vi "Inspect omv.vi"() -> ()   [LabVIEW 2013]
uses:
  <vilib>/Analysis/polynomials.llb/Unique Numbers and Multiplicity (DBL).vi
  <vilib>/Utility/file.llb/Read From Spreadsheet File (string).vi
  <vilib>/Analysis/NI_AALPro.lvlib
panel:
  in  "Open (*.omv)":path
  in  "Tab Control":enum32{"Plot", "VARS"}(tab)
  out "Waveform Graph":dbl[][](graph)
  in  "VAR":u16(ring) items=["XHV"]
  out "min":dbl
  out "max":dbl
  out "Number":i32
  out "Unique":i32
  out "Step size (average)":dbl
  out "VARS":string[](array[string])
  out "Values":string[][](array[string])
  in  "stop":bool
  # "Inspect"
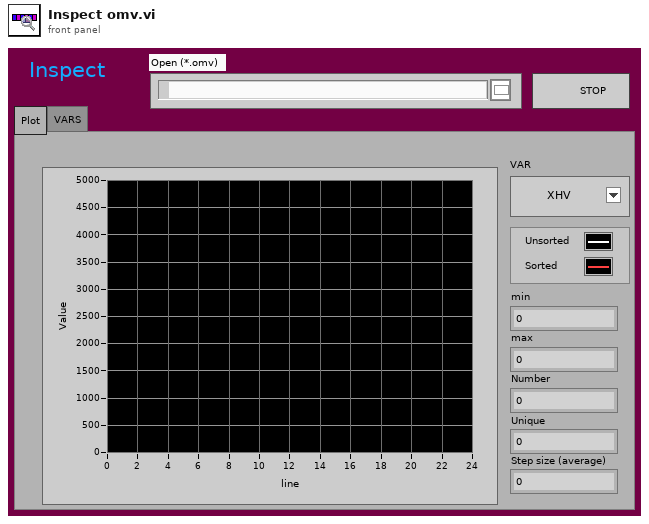
[diagram p1: front panel]
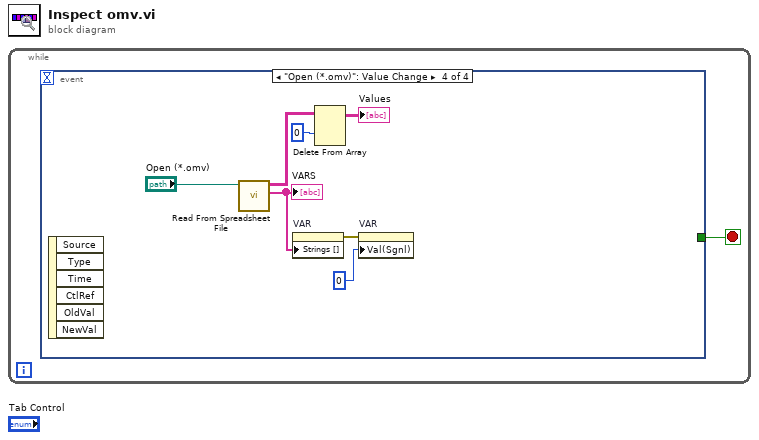
[diagram p0: block diagram]
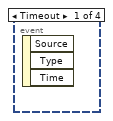
[diagram p2: hidden frame]
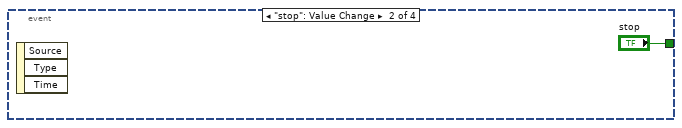
[diagram p3: hidden frame]
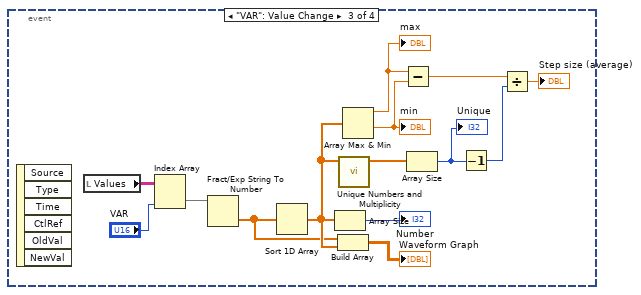
[diagram p4: hidden frame]
diagram:
  n1 = while {
    stop <- w1 stop-if-true
    n2 = event shown="[3] \"Open (*.omv)\": Value Change" {
      selector: _ -> [_ _ _ _]
      dyn-events: _ -> [_ _ _ _]
      timeout: _ -> [_ _ _ _]
      tunnel: [_ "stop" _ _] -> w1
      event Timeout {
        n3 = event-data() -> ()  [unwired: 1 in, 3 out]
      }
      event "stop": Value Change {
        n4 = event-data() -> ()  [unwired: 1 in, 3 out]
      }
      event "VAR": Value Change {
        n5 = event-data() -> ()  [unwired: 1 in, 6 out]
        n6 = local read "Values"() -> (w16:string[][])
        n7 = Index Array(array=w16, index (col)="VAR") -> (element=w3:string[])  [unwired: 1 in]
        n8 = Fract/Exp String To Number(string=w3) -> (number=w4:dbl[])  [unwired: 3 in, 1 out]
        n9 = Sort 1D Array(array=w4) -> (sorted array=w9:dbl[])
        n10 = Array Size(array=w9) -> (size(s)=→"Number":i32)
        n11 = Build Array(w4, w9) -> (→"Waveform Graph":dbl[][])
        n12 = call-poly <vilib>:"Unique Numbers and Multiplicity.vi"("Numbers"=w9) -> ("Unique Numbers"=w8:dbl[])  [unwired: 8 in, 2 out]
        n13 = Array Max & Min(array=w9) -> (max value=w13:dbl, min value=w7:dbl)  [unwired: 2 out]
        "max" <- w13
        "min" <- w7
        n14 = Subtract(x=w13, y=w7) -> (x-y=w12:dbl)
        n15 = Array Size(array=w8) -> (size(s)=w6:i32)
        "Unique" <- w6
        n16 = Decrement(x=w6) -> (x-1=w5:i32)
        n17 = Divide(x=w12, y=w5) -> (x/y=→"Step size (average)":dbl)
      }
      event "Open (*.omv)": Value Change {
        n18 = event-data() -> ()  [unwired: 1 in, 6 out]
        n19 = call-poly <vilib>:"Read From Spreadsheet File.vi"("file path (dialog if empty)"="Open (*.omv)") -> ("first row"=w20:string[], "all rows"=w22:string[][])  [unwired: 6 in, 3 out]
        "VARS" <- w20
        n20 = property on="VAR" class="Ring (strict)"("Strings []"=w20) -> (error out=w18:errorcluster)  [unwired: 2 in, 1 out]
        n21 = Delete From Array(array=w22, index (row)=0) -> (array with subset deleted=→"Values":string[][])  [unwired: 2 in, 1 out]
        n22 = property on="VAR" class="Ring (strict)"(error in=w18, "Val(Sgnl)"=u16 0 ("Value (Signaling)")) -> ()  [unwired: 1 in, 2 out]
      }
    }
  }
